vi "Queue Array Create.vi"(8 "error in (no error)":errorcluster, 10 "max queue size(-1)":i32, 11 "queue name in":string[](array[string])) -> (0 "error out":errorcluster, 1 "create new？":bool[](array[boolean]), 2 "queue out":refnum<queue>[](array[refnum]), 3 "queue name out":string[](array[string]))   [LabVIEW 2020]
uses:
  Control/Queue Data.ctl
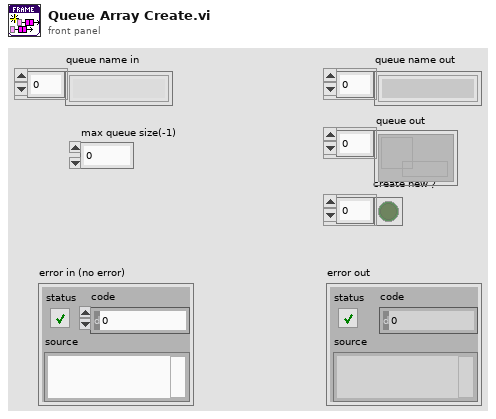
[diagram p1: front panel]
types:
  T1 = typedef "Queue Data.ctl" = cluster{"event":string, "data":variant}
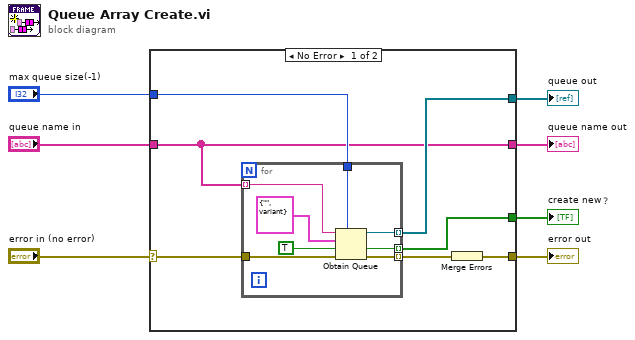
[diagram p0: block diagram]
diagram:
  n1 = case shown="No Error" "error in (no error)" {
    selector: "error in (no error)" -> [w10 w24]
    tunnel: [w8 w24] -> w6
    tunnel: "queue name in" -> [w11 w23]
    tunnel: "max queue size(-1)" -> [w14 _]
    tunnel: [w11 w23] -> w3
    tunnel: [w13 _] -> w2
    tunnel: [w12 _] -> w1
    frame No Error {
      n2 = for {
        tunnel: w14 -> [w20]
        tunnel: [w19] -> w13 mode=indexing
        tunnel: [w18] -> w12 mode=indexing
        tunnel: w11 -> [w17] mode=indexing
        tunnel: w10 -> [w16]
        tunnel: [w15] -> w9 mode=indexing
        n3 = Obtain Queue(max queue size (-1, unlimited)=w20, name (unnamed)=w17, element data type=T1 {"event"="", "data"=variant}, create if not found? (T)=TRUE, error in (no error)=w16) -> (queue out=w18:refnum<queue>, created new?=w19:bool, error out=w15:errorcluster)
      }
      n4 = Merge Errors(w9) -> (w8:errorcluster)
    }
    frame Error {
    }
  }
  "error out" <- w6
  "create new？" <- w2
  "queue name out" <- w3
  "queue out" <- w1
